vi "Newmark-Initialize.vi"(0 "VISA resource name":refnum<visa-resource-name>, 2 "ActiveStages":string[](array[string]), 5 "baud rate":u32=9600, 9 "Timeout":u32=10000, 11 "Bool Refnum":refnum<vi>) -> (4 "VISA resource name out":refnum<visa-resource-name>, 8 "Error?":bool, 15 "Error OUT":errorcluster)   [LabVIEW 2019]
uses:
  <vilib>/Instr/_visa.llb/VISA Configure Serial Port (Instr).vi
  Comm/SerialCommError.vi
panel:
  in  "Error IN":errorcluster
  out "Communication":string
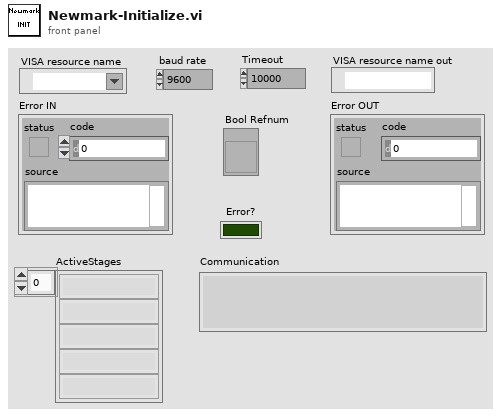
[diagram p1: front panel]
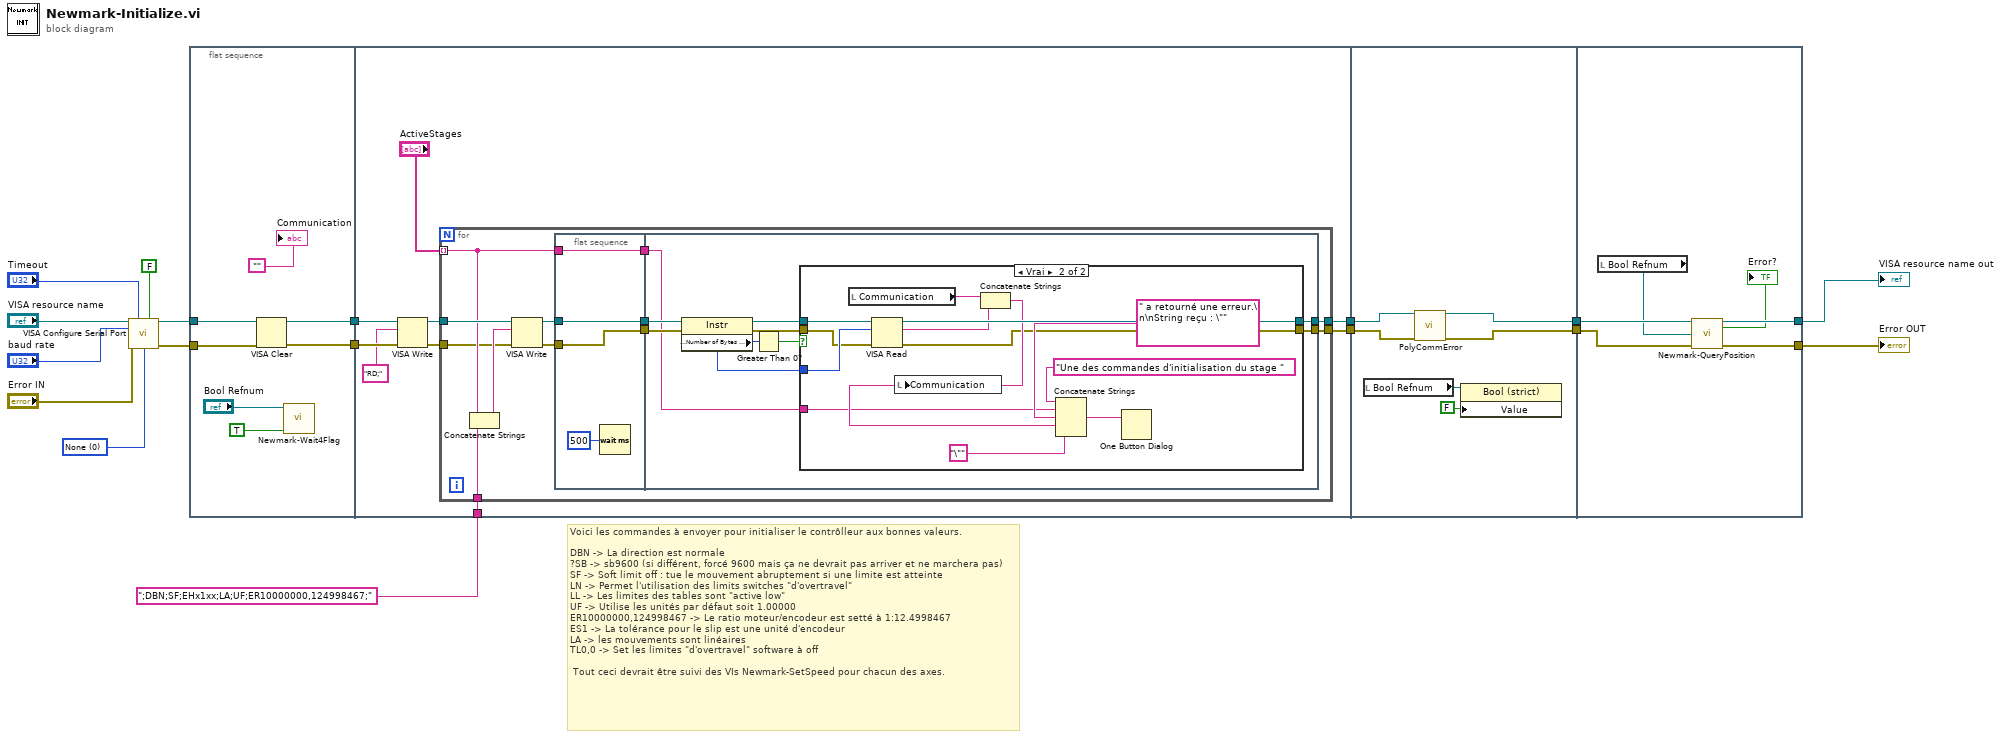
[diagram p0: block diagram]
diagram:
  w1 = u16 0 items=["None", "XON/XOFF", "RTS/CTS", "XON/XOFF & RTS/CTS", "DTR/DSR", "XON/XOFF & DTR/DSR"] ("flow control (0:none)")
  # "Voici les commandes à envoyer pour initialiser le contrôlleur aux bonnes valeurs.\n\nDBN -> La direction est normale\n?SB -> sb9600 (si différent, forcé 9600 mais ça ne devrait pas arriver et ne marchera pas)\nSF -> Soft limit off : tue le mouvement abruptement si une limite est atteinte\nLN -> Permet l'utilisation des limits switches \"d'overtravel\"\nLL -> Les limites des tables sont \"active low\"\nUF -> Utilise les unités par défaut soit 1.00000\nER10000000,124998467 -> Le ratio moteur/encodeur est setté à 1:12.4998467\nES1 -> La tolérance pour le slip est une unité d'encodeur\nLA -> les mouvements sont linéaires\nTL0,0 -> Set les limites \"d'overtravel\" software à off\n\n Tout ceci devrait être suivi des VIs Newmark-SetSpeed pour chacun des axes."
  n1 = call-poly "VISA Configure Serial Port"("VISA resource name"="VISA resource name", "timeout (10sec)"="Timeout", "Enable Termination\nChar (T)"=FALSE ("Enable Termination\nChar (T)"), "baud rate (9600)"="baud rate", "error in (no error)"="Error IN", "flow control (0:none)"=w1) -> ("VISA resource name out"=w13:refnum<visa-resource-name>, "error out"=w12:errorcluster)  [unwired: 8 in]
  n2 = flat-sequence {
    tunnel: w12 -> [w23]
    tunnel: w13 -> [w24]
    tunnel: [w22] -> w10
    tunnel: [w20] -> w8
    tunnel: ";DBN;SF;EHx1xx;LA;UF;ER10000000,124998467;" -> [w33]
    tunnel: w10 -> [w29]
    tunnel: w8 -> [w26]
    tunnel: [w32] -> w5
    tunnel: [w31] -> w3
    tunnel: w5 -> [w79]
    tunnel: [w77] -> w4
    tunnel: w3 -> [w78]
    tunnel: [w76] -> w2
    tunnel: [w82] -> w6
    tunnel: [w83] -> w9
    tunnel: w4 -> [w85]
    tunnel: w2 -> [w84]
    frame #0 {
      n3 = VISA Clear(VISA resource name=w24, error in (no error)=w23) -> (VISA resource name out=w22:refnum<visa-resource-name>, error out=w20:errorcluster)
      n4 = call "Newmark-Wait4Flag.vi"("Raise Flag ?"=TRUE ("Value"), "Ctl Refnum IN"="Bool Refnum") -> ()  [unwired: 8 in, 2 out]
      "Communication" <- ""
    }
    frame #1 {
      n5 = VISA Write(VISA resource name=w29, write buffer="RD;", error in (no error)=w26) -> (VISA resource name out=w28:refnum<visa-resource-name>, error out=w27:errorcluster)  [unwired: 1 out]
      n6 = for {
        tunnel: "ActiveStages" -> [w38] mode=indexing
        tunnel: w33 -> [w45]
        tunnel: w28 -> [w44]
        tunnel: [w36] -> w32
        tunnel: w27 -> [w35]
        tunnel: [w34] -> w31
        n7 = Concatenate Strings(w38, w45) -> (w43:string)
        n8 = VISA Write(VISA resource name=w44, write buffer=w43, error in (no error)=w35) -> (VISA resource name out=w42:refnum<visa-resource-name>, error out=w39:errorcluster)  [unwired: 1 out]
        n9 = flat-sequence {
          tunnel: w42 -> [w48]
          tunnel: [w48] -> w41
          tunnel: [w47] -> w40
          tunnel: w39 -> [w47]
          tunnel: w38 -> [w46]
          tunnel: [w46] -> w37
          tunnel: w41 -> [w58]
          tunnel: w40 -> [w57]
          tunnel: w37 -> [w53]
          tunnel: [w52] -> w36
          tunnel: [w50] -> w34
          frame #0 {
            n10 = Wait (ms)(milliseconds to wait=u32 500) -> ()  [unwired: 1 out]
          }
          frame #1 {
            n11 = property class="Instr"(reference=w58, error in=w57) -> (reference out=w56:refnum<visa-resource-name>, error out=w51:errorcluster, "Serial Settings:Number of Bytes at Serial Port"=w55:u32)
            n12 = Greater Than 0?(x=w55) -> (x > 0?=w54:bool)
            n13 = case shown="Vrai" w54 {
              tunnel: w56 -> [w60 w73]
              tunnel: [w60 w71] -> w52
              tunnel: w55 -> [_ w72]
              tunnel: w53 -> [_ w63]
              tunnel: w51 -> [w59 w62]
              tunnel: [w59 w61] -> w50
              frame False {
              }
              frame True {
                n14 = local read "Communication"() -> (w69:string)
                n15 = VISA Read(VISA resource name=w73, byte count=w72, error in (no error)=w62) -> (VISA resource name out=w71:refnum<visa-resource-name>, read buffer=w70:string, error out=w61:errorcluster)  [unwired: 1 out]
                n16 = Concatenate Strings(w69, w70) -> (w68:string)
                n17 = local write "Communication"(w68) -> ()
                n18 = Concatenate Strings("Une des commandes d'initialisation du stage " ("message"), w63, " a retourné une erreur.\n\nString reçu : \"" ("message"), w68, "\"" ("message")) -> (w67:string)
                n19 = One Button Dialog(message=w67) -> ()  [unwired: 1 in, 1 out]
              }
            }
          }
        }
      }
    }
    frame #2 {
      n20 = local read "Bool Refnum"() -> (w75:refnum<vi>)
      n21 = call-poly "PolyCommError.vi"("VISA IN"=w79, "error IN"=w78) -> ("VISA OUT"=w77:refnum<visa-resource-name>, "error OUT"=w76:errorcluster)  [unwired: 11 in, 1 out]
      n22 = property class="Bool (strict)"(reference=w75, "Value"=FALSE) -> ()  [unwired: 1 in, 2 out]
    }
    frame #3 {
      n23 = local read "Bool Refnum"() -> (w80:refnum<vi>)
      n24 = call "Newmark-QueryPosition.vi"("Table VRN IN"=w85, "Bool Refnum"=w80, "Error IN"=w84) -> ("Table VRN OUT"=w83:refnum<visa-resource-name>, "Error?"=→"Error?":bool, "Error OUT"=w82:errorcluster)  [unwired: 5 in, 5 out]
    }
  }
  "VISA resource name out" <- w9
  "Error OUT" <- w6
